vi "Cursor Page.vi"() -> ()   [LabVIEW 2020, in "3D Plot.lvclass"]
uses:
  <vilib>/Math Plots/3D Math Plots/3D Plot/3D Plot/3D Plot.lvclass
  <vilib>/Math Plots/3D Math Plots/3D Plot/3D Plot/Typedef/Cursor Property Array.ctl
  <vilib>/Math Plots/3D Math Plots/3D Plot/3D Plot/Typedef/Cursor Property.ctl
  <vilib>/Math Plots/3D Math Plots/3D Plot/3D Plot/Typedef/Cursor Position.ctl
  <vilib>/Math Plots/3D Math Plots/3D Plot/3D Plot/Typedef/Cursor Point.ctl
  <vilib>/Math Plots/3D Math Plots/3D Plot/3D Plot/Typedef/Sprite Type.ctl
  <vilib>/Math Plots/3D Math Plots/3D Plot/3D Plot/Typedef/Cursor Line.ctl
  <vilib>/Math Plots/3D Math Plots/3D Plot/3D Plot/Typedef/Line Type.ctl
  <vilib>/Math Plots/3D Math Plots/3D Plot/3D Plot/Typedef/Cursor Plane.ctl
  <vilib>/Math Plots/3D Math Plots/3D Plot/3D Plot/Typedef/Cursor Text.ctl
  <vilib>/Math Plots/3D Math Plots/3D Plot/3D Plot/Typedef/Dialog State.ctl
  <vilib>/Math Plots/3D Math Plots/3D Plot/3D Plot/Typedef/Temp Scene State.ctl
  <vilib>/Math Plots/3D Math Plots/3D Plot/3D Plot/Typedef/Temp Scene Property Action.ctl
panel:
  in  "Cursor Name":string="Cursor"
  in  "Plot ID":u16(ring) items=["Plot-1"]
  in  "Name Color":u32(colorbox) caption="Color"
  in  "Background Color":u32(colorbox) caption="Background color"
  in  "Name":u16=1 caption="Size" min=1 step=1
  in  "Show Position":bool caption="Show position"
  in  "Show Name":bool caption="Show name"
  in  "Background Opacity":sgl(slide) caption="Background opacity(%)" min=0 max=100 scale=0.0..100.0
  in  "XY Plane Visible":bool caption="XY plane visible"
  in  "XZ Plane Visible":bool caption="XZ plane visible"
  in  "YZ Plane Visible":bool caption="YZ plane visible"
  in  "Plane Color":u32(colorbox) caption="Plane color"
  in  "Plane Opacity":sgl(slide) caption="Plane opacity(%)" min=0 max=100 scale=0.0..100.0
  in  "X Position":sgl caption="X position"
  in  "Z Position":sgl caption="Z position"
  in  "Y Position":sgl caption="Y position"
  in  "Lock Style":u16(ring) caption="Lock style" items=["Fixed", "Nearest Plot", "Snap to Plot"]
  in  "Cursor Visible":bool caption="Cursor visible"
  in  "Cursor Enable":bool caption="Cursor enable"
  in  "Line Style":u16(ring) caption="Line style"
  in  "Line Color":u32(colorbox) caption="Line color"
  in  "Line Width":sgl=0.001 caption="Line width" min=0.001 step=1
  in  "Point Style":u16(ring) caption="Point style"
  in  "Point Size":sgl=0.001 caption="Point size" min=0.001 step=1
  in  "Point Color":u32(colorbox) caption="Point color"
  in  "Cursor List":i32(listbox) caption="Cursor list"
  in  "New":bool
  in  "Delete":bool
  in  "Move Up":bool caption="Move up"
  in  "Move Down":bool caption="Move down"
  out "Cursor Property Array Out":T1
  in  "Cursor Property Array In":T1
  in  "Event Registration":refnum<event-registration>
  # "Cursor"
  # "Cursor Point"
  # "Cursor Line"
  # "Cursor General"
  # "Cursor Plane"
  # "Cursor Text"
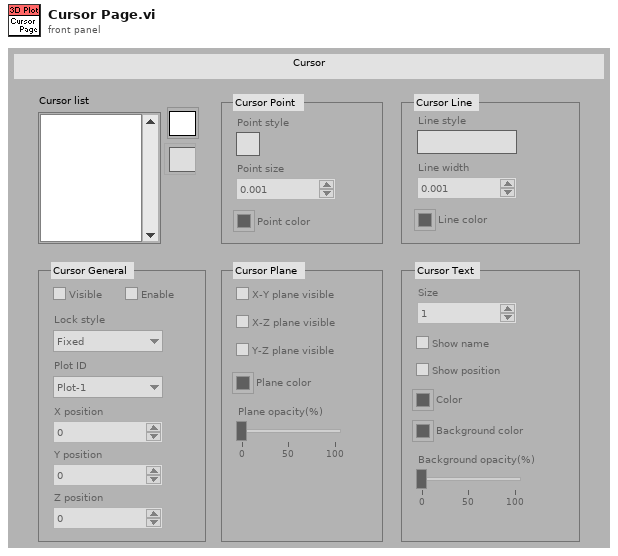
[diagram p1: front panel]
types:
  T1 = typedef "3D Plot.lvclass/Cursor Property Array.ctl" = T2[]
  T2 = typedef "3D Plot.lvclass/Cursor Property.ctl" = cluster{"Cursor Visible":bool, "Cursor Enable":bool, "Cursor Position":T3, "Cursor Point":T4, "Cursor Line":T6, "Cursor Plane":T8, "Cursor Text":T9}
  T3 = typedef "3D Plot.lvclass/Cursor Position.ctl" = cluster{"Cursor Plot ID":i32, "Cursor X":sgl, "Cursor Y":sgl, "Cursor Z":sgl, "Cursor Snap To":enum16{"Fixed", "Nearest Plot", "Snap to Plot"}}
  T4 = typedef "3D Plot.lvclass/Cursor Point.ctl" = cluster{"Cursor Point Color":u32, "Cursor Point Size":sgl, "Cursor Point Style":T5}
  T5 = typedef "3D Plot.lvclass/Sprite Type.ctl" = enum16{"None", "Empty Square", "Solid Square", "Empty Diamond", "Solid Diamond", "Empty Circle", "Solid Circle", "Asterisk", "Bold X", "Wireframe Sphere", "Solid Sphere", "Wireframe Cube", "Solid Cube"}
  T6 = typedef "3D Plot.lvclass/Cursor Line.ctl" = cluster{"Cursor Line Color":u32, "Cursor Line Width":sgl, "Cursor Line Style":T7}
  T7 = typedef "3D Plot.lvclass/Line Type.ctl" = enum16{"None", "Solid", "Dash", "Dot", "Dash Dot"}
  T8 = typedef "3D Plot.lvclass/Cursor Plane.ctl" = cluster{"Cursor Plane Color":u32, "Cursor Plane Opacity":sgl, "Draw Cursor Plane X-Z":bool, "Draw Cursor Plane Y-Z":bool, "Draw Cursor Plane X-Y":bool}
  T9 = typedef "3D Plot.lvclass/Cursor Text.ctl" = cluster{"Cursor Text":string, "Cursor Text Size":u16, "Cursor Show Position":bool, "Cursor Show Name":bool, "Cursor Text Color":u32, "Background Color":u32, "Background Opacity":sgl}
  T10 = typedef "3D Plot.lvclass/Dialog State.ctl" = enum16{"Initialize", "Read Porperty", "Write Property", "Idle", "Exit"}
  T11 = typedef "3D Plot.lvclass/Temp Scene Property Action.ctl" = enum16{"Graph Property", "Light Property", "Axis Property", "Value Pair Property", "Format Property", "Cursor Property", "Plot Specific Property"}
  T12 = typedef "3D Plot.lvclass/Temp Scene State.ctl" = enum16{"Create", "Update Scene", "Get Plot Representation", "Destory"}
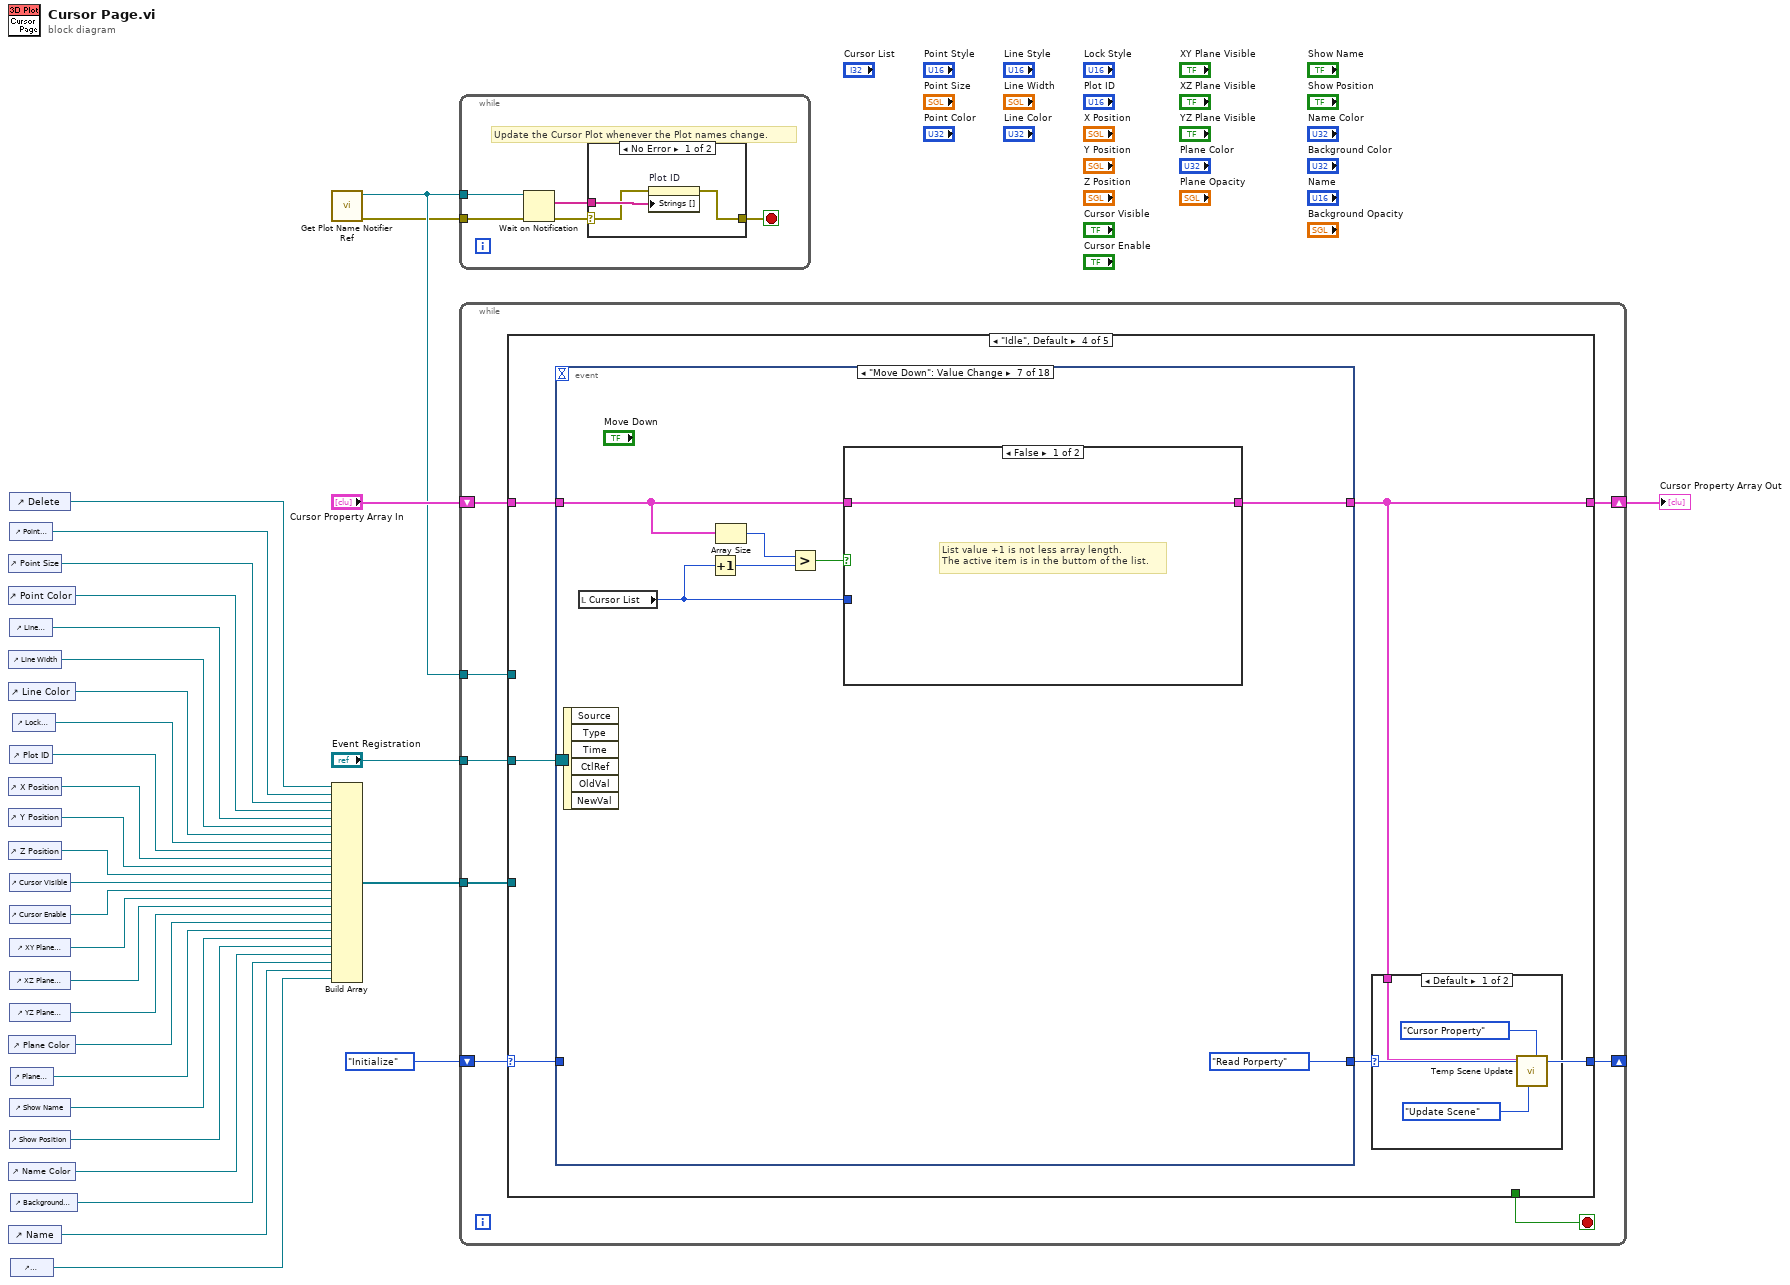
[diagram p0: block diagram]
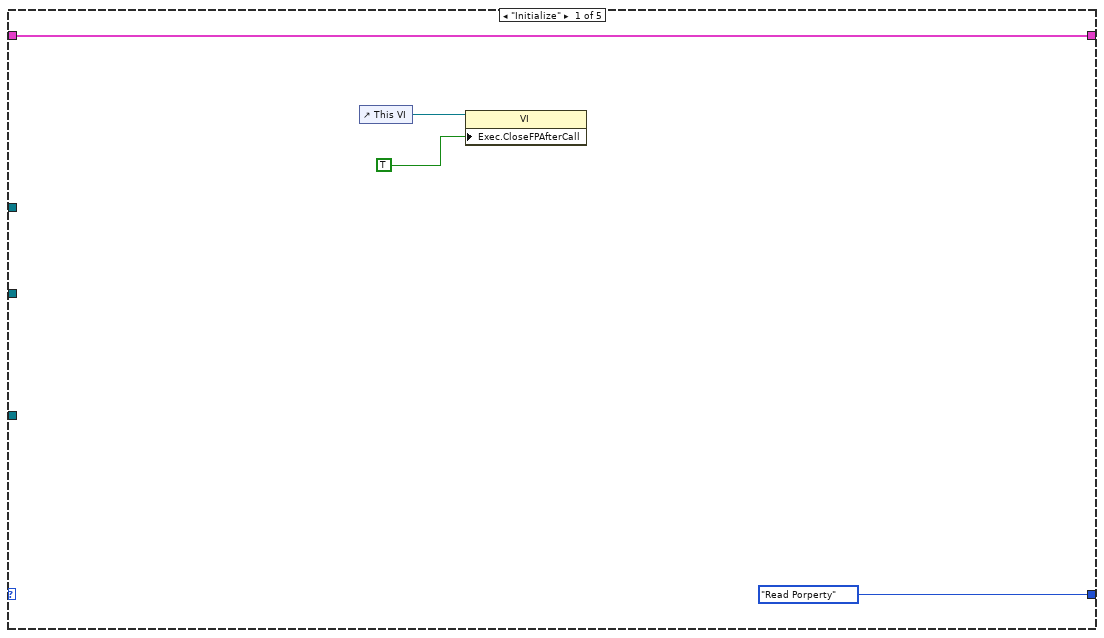
[diagram p3: hidden frame]
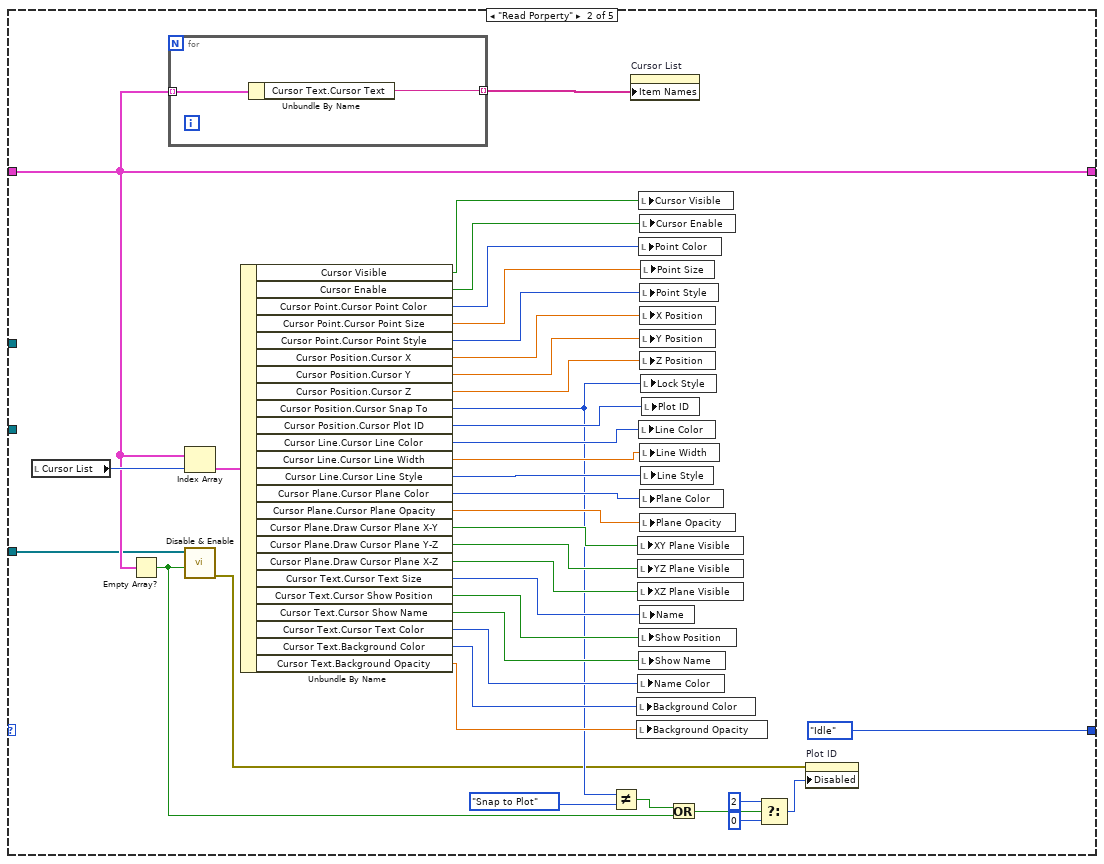
[diagram p4: hidden frame]
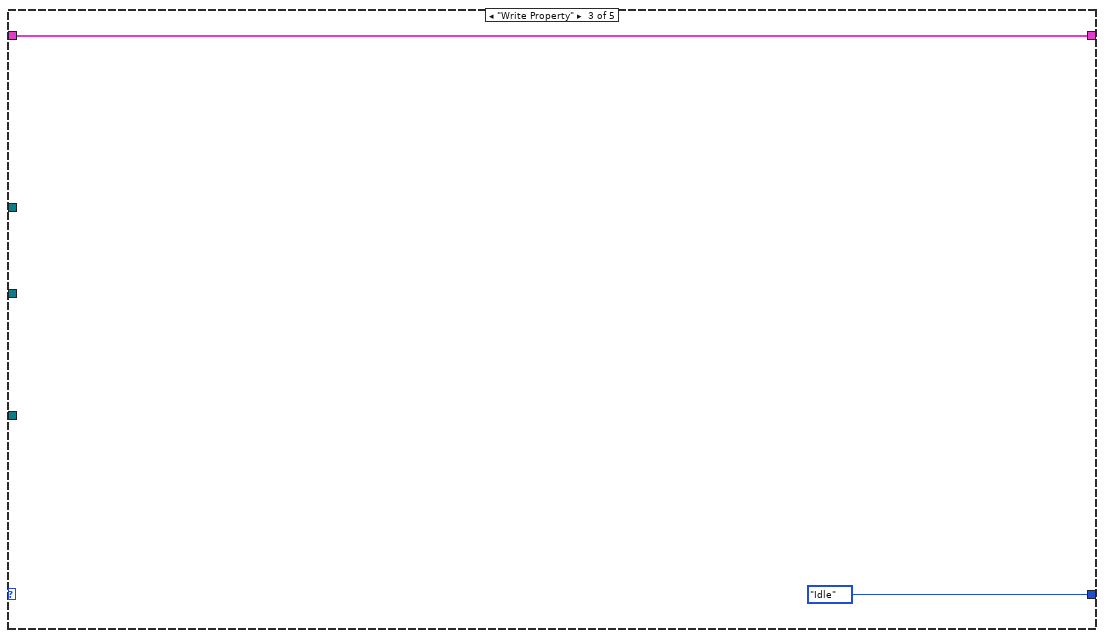
[diagram p5: hidden frame]
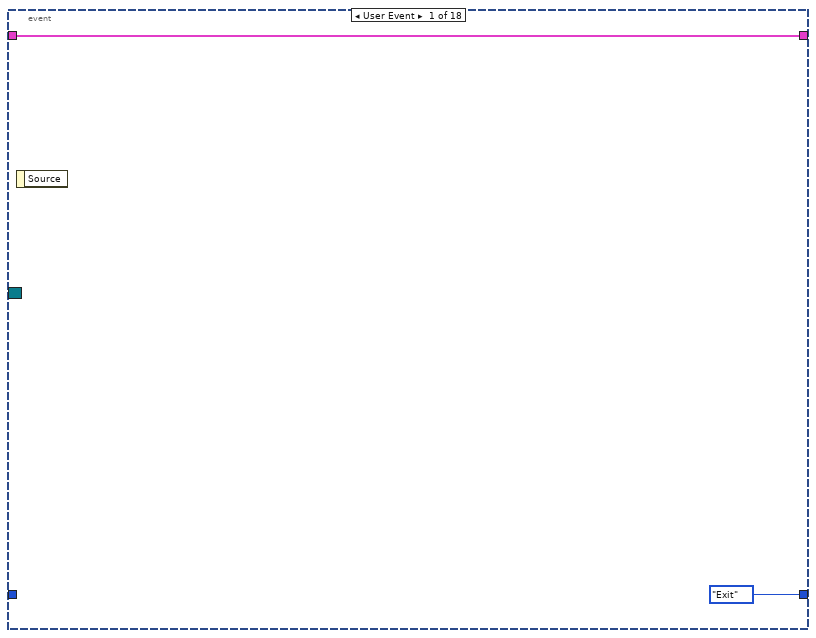
[diagram p7: hidden frame]
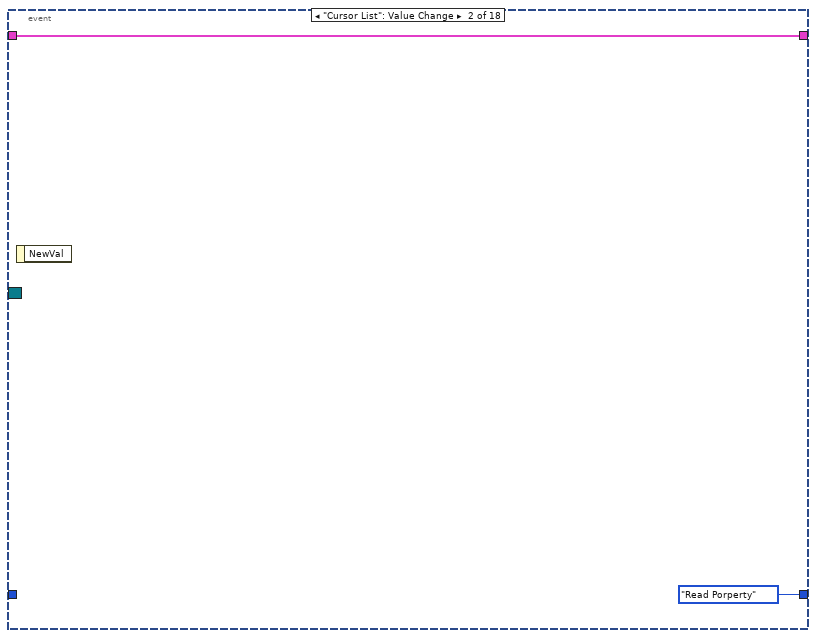
[diagram p8: hidden frame]
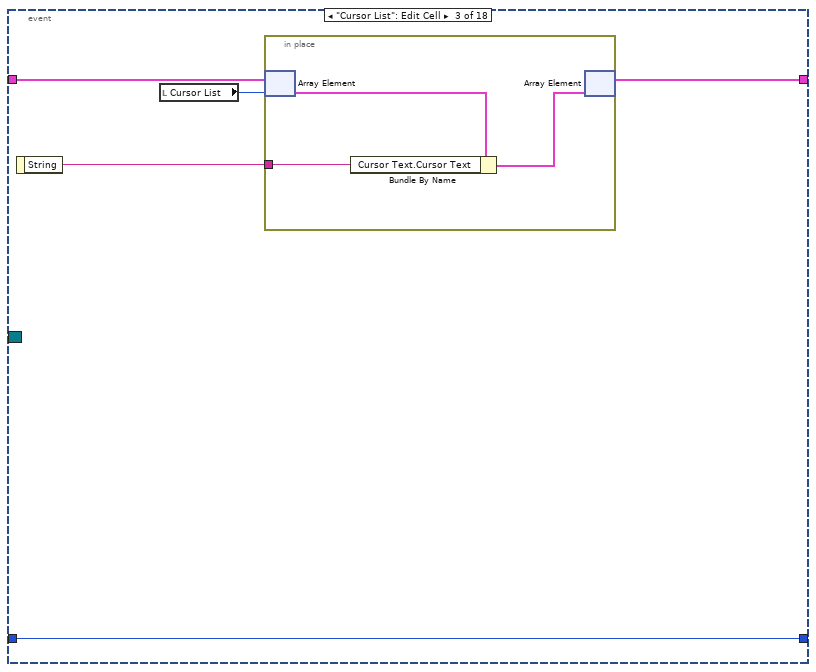
[diagram p9: hidden frame]
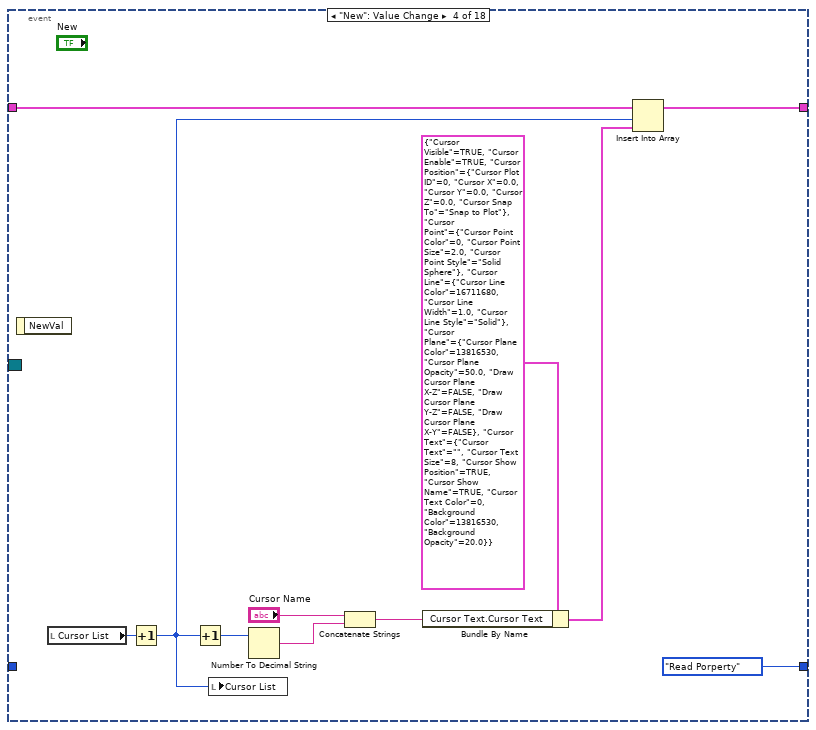
[diagram p10: hidden frame]
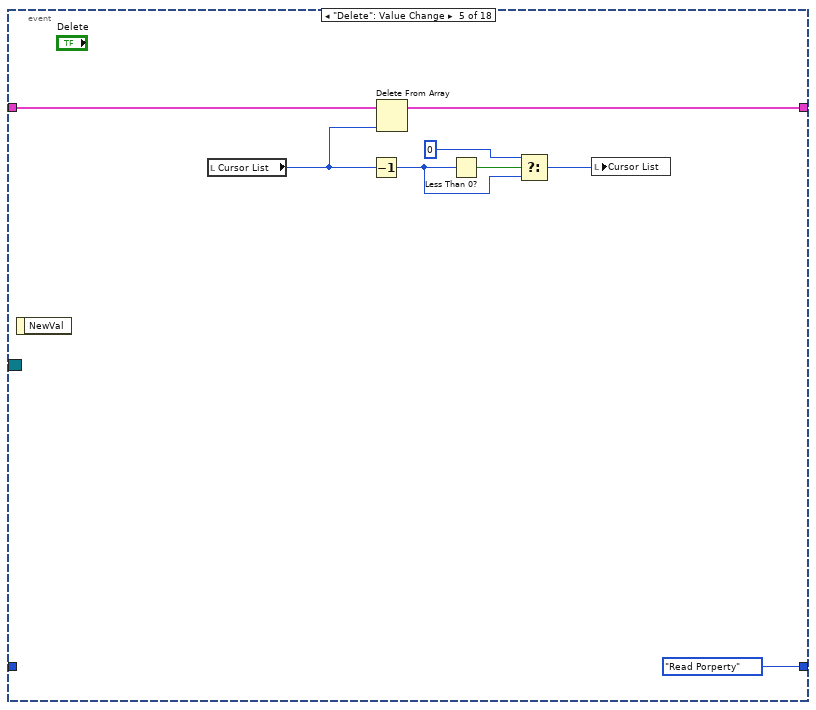
[diagram p11: hidden frame]
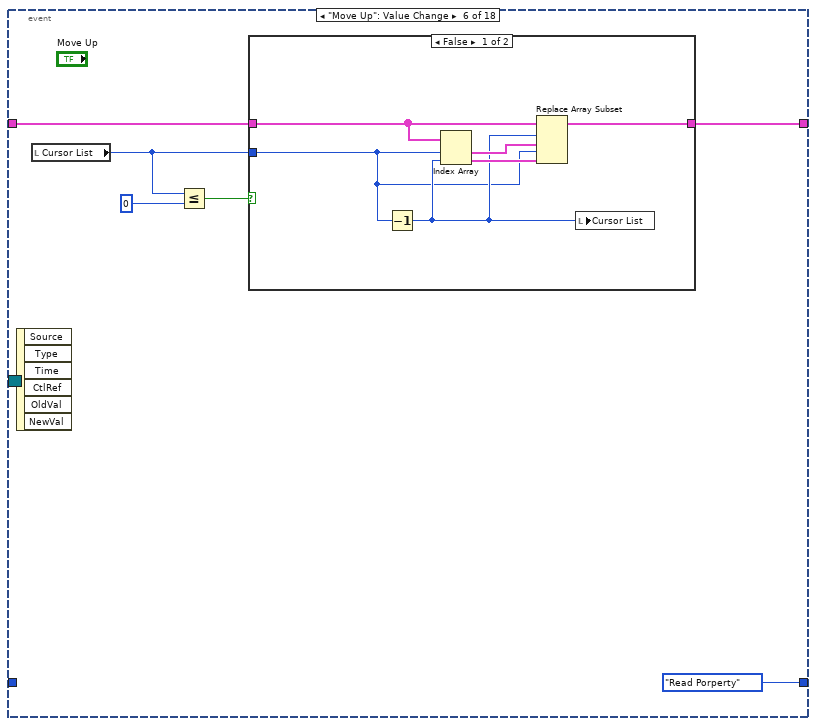
[diagram p12: hidden frame]
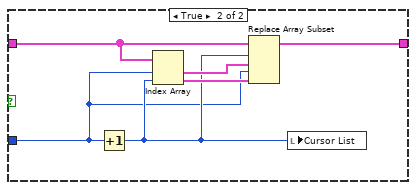
[diagram p14: hidden frame]
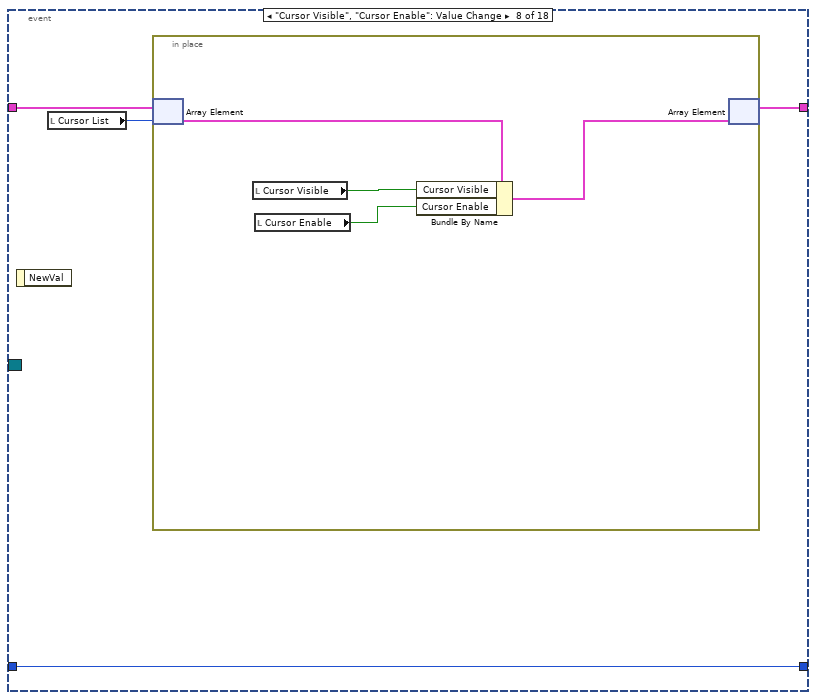
[diagram p15: hidden frame]
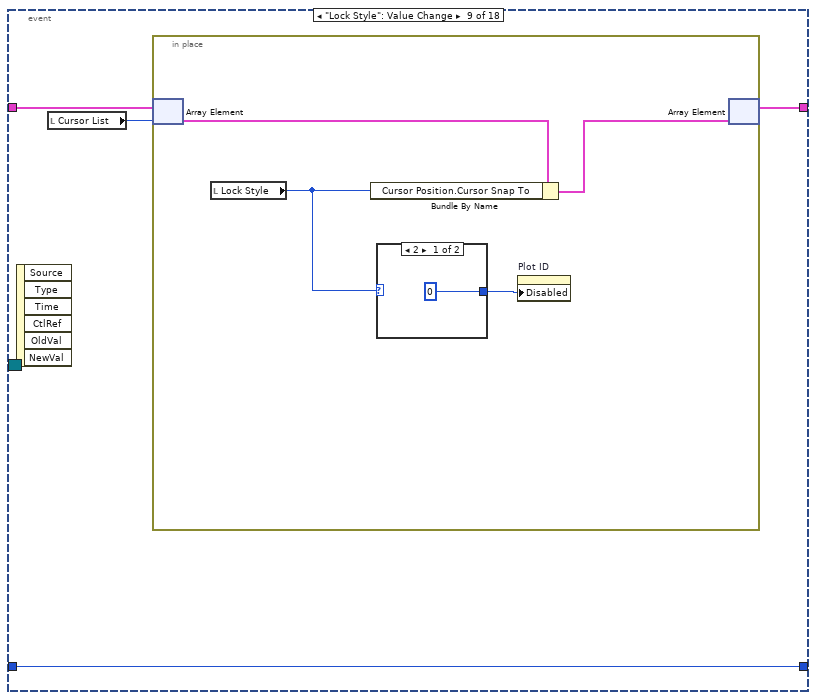
[diagram p16: hidden frame]
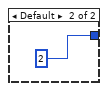
[diagram p17: hidden frame]
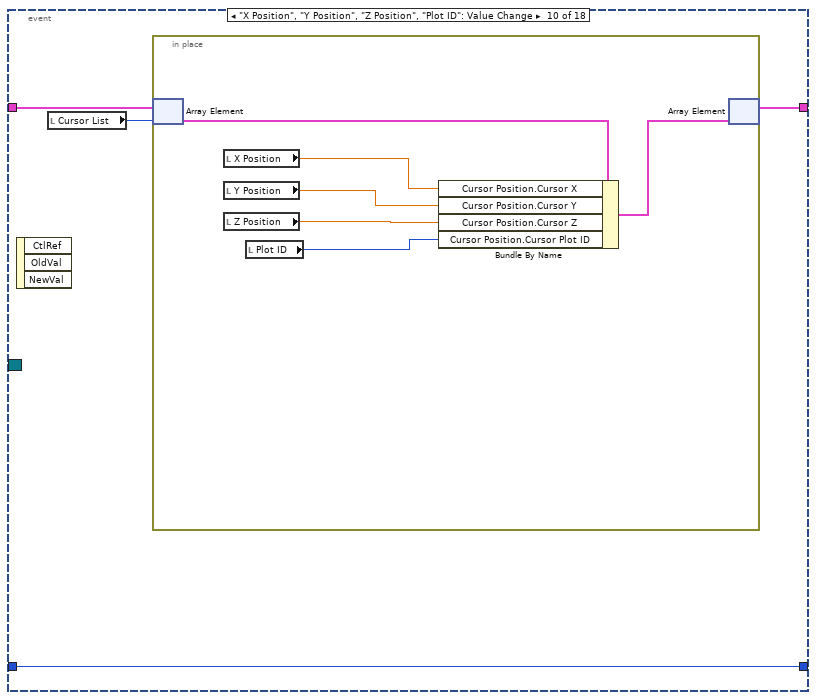
[diagram p18: hidden frame]
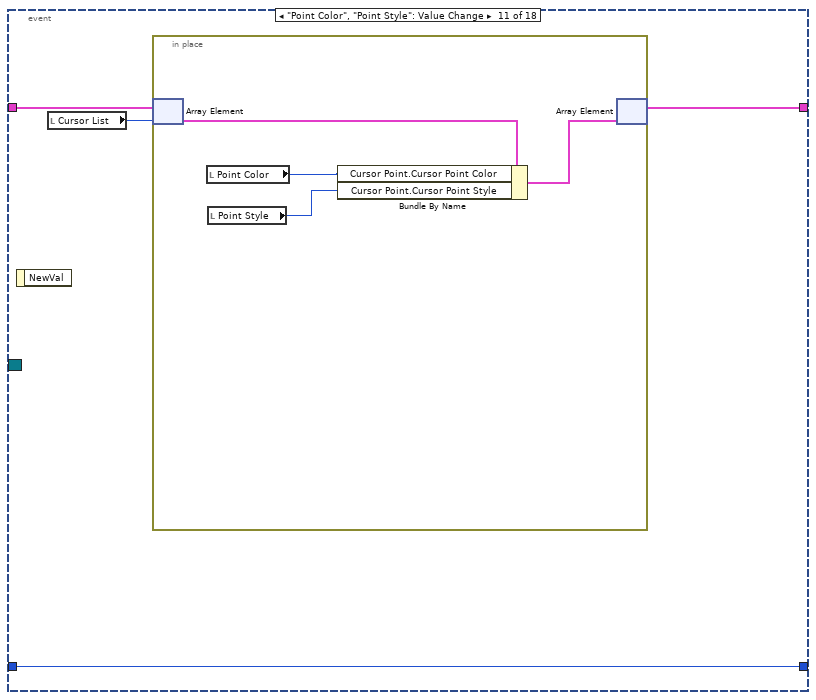
[diagram p19: hidden frame]
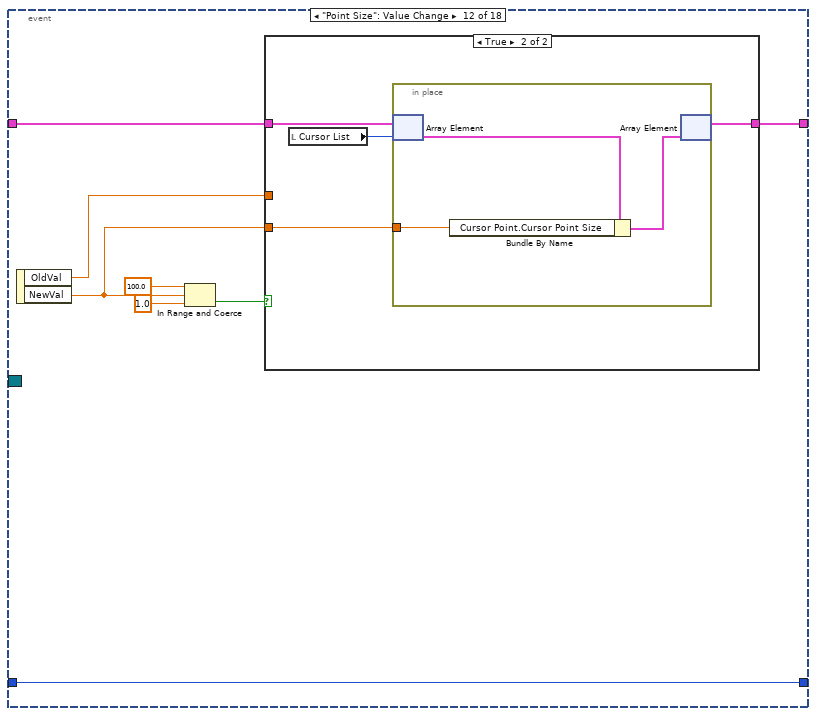
[diagram p20: hidden frame]
diagram:
  n1 = control-ref of="Point Size"() -> (w25:refnum<vi>)
  n2 = control-ref of="Point Color"() -> (w24:refnum<vi>)
  n3 = control-ref of="Line Width"() -> (w22:refnum<vi>)
  n4 = control-ref of="Line Color"() -> (w21:refnum<vi>)
  n5 = control-ref of="X Position"() -> (w18:refnum<vi>)
  n6 = control-ref of="Y Position"() -> (w17:refnum<vi>)
  n7 = control-ref of="Z Position"() -> (w16:refnum<vi>)
  n8 = control-ref of="Plane Color"() -> (w10:refnum<vi>)
  n9 = control-ref of="Name Color"() -> (w7:refnum<vi>)
  n10 = control-ref of="Name"() -> (w5:refnum<vi>)
  n11 = control-ref of="Delete"() -> (w1:refnum<vi>)
  n12 = control-ref of="Point Style"() -> (w26:refnum<vi>)
  n13 = control-ref of="Line Style"() -> (w23:refnum<vi>)
  n14 = control-ref of="Plot ID"() -> (w19:refnum<vi>)
  n15 = control-ref of="Cursor Visible"() -> (w15:refnum<vi>)
  n16 = control-ref of="Cursor Enable"() -> (w14:refnum<vi>)
  n17 = control-ref of="XY Plane Visible"() -> (w13:refnum<vi>)
  n18 = control-ref of="XZ Plane Visible"() -> (w12:refnum<vi>)
  n19 = control-ref of="YZ Plane Visible"() -> (w11:refnum<vi>)
  n20 = control-ref of="Show Name"() -> (w9:refnum<vi>)
  n21 = control-ref of="Show Position"() -> (w8:refnum<vi>)
  n22 = control-ref of="Plane Opacity"() -> (w3:refnum<vi>)
  n23 = control-ref of="Background Color"() -> (w6:refnum<vi>)
  n24 = control-ref of="Background Opacity"() -> (w4:refnum<vi>)
  n25 = control-ref of="Lock Style"() -> (w20:refnum<vi>)
  n26 = call <vilib>:"Get Plot Name Notifier Ref.vi"() -> ("error out"=w27:errorcluster, "Plot Names Notifier Ref"=w28:refnum<notifier>)  [unwired: 1 in, 9 out]
  n27 = Build Array(w1, w26, w25, w24, w23, w22, w21, w20, w19, w18, w17, w16, w15, w14, w13, w12, w11, w10, w3, w9, w8, w7, w6, w5, w4) -> (w2:refnum<vi>[])
  n28 = while {
    tunnel: w28 -> [w37]
    tunnel: w27 -> [w33]
    stop <- w34 stop-if-true
    # "Update the Cursor Plot whenever the Plot names change."
    n29 = Wait on Notification(notifier=w37, error in (no error)=w33) -> (notification=w36:string[], error out=w35:errorcluster)  [unwired: 4 out]
    n30 = case shown="No Error" w35 {
      selector: w35 -> [w39 w41]
      tunnel: w36 -> [w40 _]
      tunnel: [w38 w41] -> w34
      frame No Error {
        n31 = property on="Plot ID" class="Ring (strict)"(error in=w39, "Strings []"=w40) -> (error out=w38:errorcluster)  [unwired: 1 in, 1 out]
      }
      frame Error {
      }
    }
  }
  n32 = while {
    shift-right: [w48] -> w32
    shift-left: "Cursor Property Array In" -> [w49]
    shift-right: [w44] -> _
    shift-left: Dialog_State."Initialize" -> [w47]
    tunnel: "Event Registration" -> [w45]
    tunnel: w28 -> [w43]
    tunnel: w2 -> [w42]
    stop <- w46 stop-if-true
    n33 = case shown="\"Idle\", Default" w47 {
      selector: w47 -> [_ _ _ w98 _]
      tunnel: w49 -> [w52 w64 w94 w100 w279]
      tunnel: [w52 w64 w94 w97 w279] -> w48
      tunnel: [Dialog_State."Read Porperty" Dialog_State."Idle" Dialog_State."Idle" w96 Dialog_State."Exit"] -> w44
      tunnel: [_ _ _ _ TRUE] -> w46
      tunnel: w45 -> [_ _ _ w99 _]
      tunnel: w43 -> [_ _ _ _ w278]
      tunnel: w42 -> [_ w63 _ _ _]
      frame "Initialize" {
        n34 = control-ref of="This VI"() -> (w51:refnum<vi>)
        n35 = property class="VI"(reference=w51, "Exec.CloseFPAfterCall"=TRUE ("Execution:Close After Call")) -> ()  [unwired: 1 in, 2 out]
      }
      frame "Read Porperty" {
        n36 = local read "Cursor List"() -> (w66:i32)
        n37 = Empty Array?(array=w64) -> (empty?=w59:bool)
        n38 = for {
          tunnel: w64 -> [w93] mode=indexing
          tunnel: [w92] -> w67 mode=indexing
          n39 = Unbundle By Name(w93) -> ("Cursor Text.Cursor Text"=w92:string)
        }
        n40 = Index Array(array=w64, index=w66) -> (element=w90:T2)
        n41 = call <vilib>:"Disable & Enable.vi"("Disabled?"=w59, "Control Ref Array"=w63) -> ("error out"=w54:errorcluster)  [unwired: 1 in, 8 out]
        n42 = Unbundle By Name(w90) -> ("Cursor Visible"=w89:bool, "Cursor Enable"=w88:bool, "Cursor Point.Cursor Point Color"=w87:u32, "Cursor Point.Cursor Point Size"=w86:sgl, "Cursor Point.Cursor Point Style"=w85:T5, "Cursor Position.Cursor X"=w84:sgl, "Cursor Position.Cursor Y"=w83:sgl, "Cursor Position.Cursor Z"=w82:sgl, "Cursor Position.Cursor Snap To"=w61:enum16{"Fixed", "Nearest Plot", "Snap to Plot"}, "Cursor Position.Cursor Plot ID"=w65:i32, "Cursor Line.Cursor Line Color"=w81:u32, "Cursor Line.Cursor Line Width"=w80:sgl, "Cursor Line.Cursor Line Style"=w79:T7, "Cursor Plane.Cursor Plane Color"=w78:u32, "Cursor Plane.Cursor Plane Opacity"=w77:sgl, "Cursor Plane.Draw Cursor Plane X-Y"=w76:bool, "Cursor Plane.Draw Cursor Plane Y-Z"=w75:bool, "Cursor Plane.Draw Cursor Plane X-Z"=w74:bool, "Cursor Text.Cursor Text Size"=w70:u16, "Cursor Text.Cursor Show Position"=w72:bool, "Cursor Text.Cursor Show Name"=w73:bool, "Cursor Text.Cursor Text Color"=w69:u32, "Cursor Text.Background Color"=w71:u32, "Cursor Text.Background Opacity"=w68:sgl)
        n43 = Not Equal?(x=w61, y=enum16{"Fixed", "Nearest Plot", "Snap to Plot"}."Snap to Plot" ("Cursor Position.Cursor Snap To")) -> (x != y?=w60:bool)
        n44 = property on="Cursor List" class="LstBox (strict)"("Item Names"=w67) -> ()  [unwired: 2 in, 2 out]
        n45 = local write "Background Color"(w71) -> ()
        n46 = local write "Background Opacity"(w68) -> ()
        n47 = local write "XY Plane Visible"(w76) -> ()
        n48 = local write "YZ Plane Visible"(w75) -> ()
        n49 = local write "XZ Plane Visible"(w74) -> ()
        n50 = local write "Name Color"(w69) -> ()
        n51 = local write "Cursor Visible"(w89) -> ()
        n52 = local write "Point Color"(w87) -> ()
        n53 = local write "Line Color"(w81) -> ()
        n54 = local write "Show Position"(w72) -> ()
        n55 = local write "Show Name"(w73) -> ()
        n56 = local write "Cursor Enable"(w88) -> ()
        n57 = local write "Point Style"(w85) -> ()
        n58 = local write "X Position"(w84) -> ()
        n59 = local write "Y Position"(w83) -> ()
        n60 = local write "Z Position"(w82) -> ()
        n61 = local write "Line Width"(w80) -> ()
        n62 = local write "Plane Color"(w78) -> ()
        n63 = local write "Plane Opacity"(w77) -> ()
        n64 = local write "Name"(w70) -> ()
        n65 = local write "Point Size"(w86) -> ()
        n66 = local write "Lock Style"(w61) -> ()
        n67 = local write "Line Style"(w79) -> ()
        n68 = local write "Plot ID"(w65) -> ()
        n69 = Or(x=w60, y=w59) -> (x .or. y?=w56:bool)
        n70 = Select(t=u8 2 ("Disabled"), s=w56, f=u8 0 ("Disabled")) -> (s? t:f=w55:u8)
        n71 = property on="Plot ID" class="Ring (strict)"(error in=w54, "Disabled"=w55) -> ()  [unwired: 1 in, 2 out]
      }
      frame "Write Property" {
      }
      frame "Idle", Default {
        n72 = event shown="[6] \"Move Down\": Value Change" {
          selector: w99 -> [_ _ _ _ _ _ _ _ _ _ _ _ _ _ _ _ _ _]
          dyn-events: _ -> [_ _ _ _ _ _ _ _ _ _ _ _ _ _ _ _ _ _]
          timeout: _ -> [_ _ _ _ _ _ _ _ _ _ _ _ _ _ _ _ _ _]
          tunnel: w100 -> [w105 w107 w112 w126 w134 w140 w150 w165 w173 w182 w193 w205 w218 w227 w243 w254 w261 w273]
          tunnel: [w105 w107 w109 w125 w133 w139 w154 w164 w172 w181 w192 w204 w216 w226 w242 w253 w260 w272] -> w97
          tunnel: [Dialog_State."Exit" Dialog_State."Read Porperty" w108 Dialog_State."Read Porperty" Dialog_State."Read Porperty" Dialog_State."Read Porperty" Dialog_State."Read Porperty" w162 w170 w180 w190 w203 w215 w223 w240 w251 w258 w270] -> w96
          tunnel: w98 -> [_ _ w108 _ _ _ _ w162 w170 w180 w190 w203 w215 w223 w240 w251 w258 w270]
          event User Event {
            n73 = event-data() -> ()  [unwired: 2 out]
          }
          event "Cursor List": Value Change {
            n74 = event-data() -> ()  [unwired: 2 out]
          }
          event "Cursor List": Edit Cell {
            n75 = event-data() -> ("String"=w110:string)  [unwired: 1 out]
            n76 = local read "Cursor List"() -> (w111:i32)
            n77 = in-place {
              in-place-border: w110 -> [w113]
              n78 = in-place-array #1(w112, w111) -> (w115:T2)
              n79 = Bundle By Name(cluster=w115, "Cursor Text.Cursor Text"=w113) -> (w114:T2)
              n80 = in-place-array #1(w114) -> (w109:T1)  [unwired: 1 out]
            }
          }
          event "New": Value Change {
            n81 = event-data() -> ()  [unwired: 2 out]
            n82 = local read "Cursor List"() -> (w117:i32)
            n83 = Increment(x=w117) -> (x+1=w116:i32)
            n84 = Increment(x=w116) -> (x+1=w118:i32)
            n85 = local write "Cursor List"(w116) -> ()
            n86 = Number To Decimal String(number=w118) -> (decimal integer string=w120:string)  [unwired: 1 out]
            n87 = Concatenate Strings("Cursor Name", w120) -> (w122:string)
            n88 = Bundle By Name(cluster=T2 {"Cursor Visible"=TRUE, "Cursor Enable"=TRUE, "Cursor Position"={"Cursor Plot ID"=0, "Cursor X"=0.0, "Cursor Y"=0.0, "Cursor Z"=0.0, "Cursor Snap To"=enum."Snap to Plot"}, "Cursor Point"={"Cursor Point Color"=0, "Cursor Point Size"=2.0, "Cursor Point Style"=enum."Solid Sphere"}, "Cursor Line"={"Cursor Line Color"=16711680, "Cursor Line Width"=1.0, "Cursor Line Style"=enum."Solid"}, "Cursor Plane"={"Cursor Plane Color"=13816530, "Cursor Plane Opacity"=50.0, "Draw Cursor Plane X-Z"=FALSE, "Draw Cursor Plane Y-Z"=FALSE, "Draw Cursor Plane X-Y"=FALSE}, "Cursor Text"={"Cursor Text"="", "Cursor Text Size"=8, "Cursor Show Position"=TRUE, "Cursor Show Name"=TRUE, "Cursor Text Color"=0, "Background Color"=13816530, "Background Opacity"=20.0}} ("new element/subarray"), "Cursor Text.Cursor Text"=w122) -> (w123:T2)
            n89 = Insert Into Array(array=w126, index=w116, new element=w123) -> (w125:T1)
          }
          event "Delete": Value Change {
            n90 = event-data() -> ()  [unwired: 2 out]
            n91 = local read "Cursor List"() -> (w128:i32)
            n92 = Decrement(x=w128) -> (x-1=w129:i32)
            n93 = Delete From Array(array=w134, index=w128) -> (array with subset deleted=w133:T1)  [unwired: 1 in, 1 out]
            n94 = Less Than 0?(x=w129) -> (x < 0?=w131:bool)
            n95 = Select(t=0, s=w131, f=w129) -> (s? t:f=w127:i32)
            n96 = local write "Cursor List"(w127) -> ()
          }
          event "Move Up": Value Change {
            n97 = event-data() -> ()  [unwired: 7 out]
            n98 = local read "Cursor List"() -> (w135:i32)
            n99 = Less Or Equal?(x=w135, y=0) -> (x <= y?=w136:bool)
            n100 = case shown="False" w136 {
              tunnel: w140 -> [w144 w147]
              tunnel: [w143 w147] -> w139
              tunnel: w135 -> [w141 _]
              frame False {
                n101 = Decrement(x=w141) -> (x-1=w142:i32)
                n102 = Index Array(array=w144, index #1=w141, index #2=w142) -> (element #1=w145:T2, element #2=w146:T2)
                n103 = Replace Array Subset(array=w144, new element #1=w145, index #1=w142, new element #2=w146, index #2=w141) -> (w143:T1)
                n104 = local write "Cursor List"(w142) -> ()
              }
              frame True {
                # "List value is less or equal to 0.\nThe active item is in the top of the list."
              }
            }
          }
          event "Move Down": Value Change {
            n105 = event-data() -> ()  [unwired: 7 out]
            n106 = local read "Cursor List"() -> (w149:i32)
            n107 = Increment(x=w149) -> (x+1=w152:i32)
            n108 = Array Size(array=w150) -> (size(s)=w151:i32)
            n109 = Greater?(x=w151, y=w152) -> (0:w148:bool)
            n110 = case shown="False" w148 {
              tunnel: [w155 w159] -> w154
              tunnel: w150 -> [w155 w157]
              tunnel: w149 -> [_ w156]
              frame False {
                # "List value +1 is not less array length.\nThe active item is in the buttom of the list."
              }
              frame True {
                n111 = Increment(x=w156) -> (x+1=w158:i32)
                n112 = Index Array(array=w157, index #1=w156, index #2=w158) -> (element #1=w160:T2, element #2=w161:T2)
                n113 = Replace Array Subset(array=w157, new element #1=w160, index #1=w158, new element #2=w161, index #2=w156) -> (w159:T1)
                n114 = local write "Cursor List"(w158) -> ()
              }
            }
          }
          event "Cursor Visible", "Cursor Enable": Value Change {
            n115 = event-data() -> ()  [unwired: 2 out]
            n116 = local read "Cursor List"() -> (w163:i32)
            n117 = in-place {
              n118 = in-place-array #2(w165, w163) -> (w167:T2)
              n119 = local read "Cursor Visible"() -> (w169:bool)
              n120 = local read "Cursor Enable"() -> (w168:bool)
              n121 = Bundle By Name(cluster=w167, "Cursor Visible"=w169, "Cursor Enable"=w168) -> (w166:T2)
              n122 = in-place-array #2(w166) -> (w164:T1)  [unwired: 1 out]
            }
          }
          event "Lock Style": Value Change {
            n123 = event-data() -> ()  [unwired: 7 out]
            n124 = local read "Cursor List"() -> (w171:i32)
            n125 = in-place {
              n126 = in-place-array #3(w173, w171) -> (w177:T2)
              n127 = local read "Lock Style"() -> (w175:u16)
              n128 = Bundle By Name(cluster=w177, "Cursor Position.Cursor Snap To"=w175) -> (w176:T2)
              n129 = case shown="2" w175 {
                tunnel: [u8 0 ("Disabled") u8 2 ("Disabled")] -> w174
                frame 2 {
                }
                frame Default {
                }
              }
              n130 = property on="Plot ID" class="Ring (strict)"("Disabled"=w174) -> ()  [unwired: 2 in, 2 out]
              n131 = in-place-array #3(w176) -> (w172:T1)  [unwired: 1 out]
            }
          }
          event "X Position", "Y Position", "Z Position", "Plot ID": Value Change {
            n132 = event-data() -> ()  [unwired: 4 out]
            n133 = local read "Cursor List"() -> (w183:i32)
            n134 = in-place {
              n135 = in-place-array #4(w182, w183) -> (w189:T2)
              n136 = local read "X Position"() -> (w187:sgl)
              n137 = local read "Y Position"() -> (w186:sgl)
              n138 = local read "Z Position"() -> (w185:sgl)
              n139 = local read "Plot ID"() -> (w184:u16)
              n140 = Bundle By Name(cluster=w189, "Cursor Position.Cursor X"=w187, "Cursor Position.Cursor Y"=w186, "Cursor Position.Cursor Z"=w185, "Cursor Position.Cursor Plot ID"=w184) -> (w188:T2)
              n141 = in-place-array #4(w188) -> (w181:T1)  [unwired: 1 out]
            }
          }
          event "Point Color", "Point Style": Value Change {
            n142 = event-data() -> ()  [unwired: 2 out]
            n143 = local read "Cursor List"() -> (w191:i32)
            n144 = in-place {
              n145 = in-place-array #5(w193, w191) -> (w196:T2)
              n146 = local read "Point Color"() -> (w197:u32)
              n147 = local read "Point Style"() -> (w194:u16)
              n148 = Bundle By Name(cluster=w196, "Cursor Point.Cursor Point Color"=w197, "Cursor Point.Cursor Point Style"=w194) -> (w195:T2)
              n149 = in-place-array #5(w195) -> (w192:T1)  [unwired: 1 out]
            }
          }
          event "Point Size": Value Change {
            n150 = event-data() -> ("OldVal"=w198:sgl, "NewVal"=w199:sgl)  [unwired: 1 out]
            n151 = In Range and Coerce(upper limit=sgl 100.0, x=w199, lower limit=sgl 1.0) -> (In Range?=w200:bool)  [unwired: 1 out]
            n152 = case shown="True" w200 {
              tunnel: w205 -> [w206 w211]
              tunnel: [w206 w210] -> w204
              tunnel: w199 -> [_ w208]
              tunnel: w198 -> [w207 _]
              frame False {
                n153 = local write "Point Size"(w207) -> ()
              }
              frame True {
                n154 = local read "Cursor List"() -> (w209:i32)
                n155 = in-place {
                  in-place-border: w208 -> [w212]
                  n156 = in-place-array #6(w211, w209) -> (w214:T2)
                  n157 = Bundle By Name(cluster=w214, "Cursor Point.Cursor Point Size"=w212) -> (w213:T2)
                  n158 = in-place-array #6(w213) -> (w210:T1)  [unwired: 1 out]
                }
              }
            }
          }
          event "Line Color", "Line Style": Value Change {
            n159 = event-data() -> ()  [unwired: 2 out]
            n160 = local read "Cursor List"() -> (w217:i32)
            n161 = in-place {
              n162 = in-place-array #7(w218, w217) -> (w222:T2)
              n163 = local read "Line Color"() -> (w220:u32)
              n164 = local read "Line Style"() -> (w219:u16)
              n165 = Bundle By Name(cluster=w222, "Cursor Line.Cursor Line Color"=w220, "Cursor Line.Cursor Line Style"=w219) -> (w221:T2)
              n166 = in-place-array #7(w221) -> (w216:T1)  [unwired: 1 out]
            }
          }
          event "Line Width": Value Change {
            n167 = event-data() -> ("OldVal"=w224:sgl, "NewVal"=w225:sgl)  [unwired: 1 out]
            n168 = In Range and Coerce(upper limit=sgl 100.0, x=w225, lower limit=sgl 1.0) -> (In Range?=w228:bool)  [unwired: 1 out]
            n169 = case shown="True" w228 {
              tunnel: w227 -> [w231 w236]
              tunnel: [w231 w235] -> w226
              tunnel: w225 -> [_ w233]
              tunnel: w224 -> [w232 _]
              frame False {
                n170 = local write "Line Width"(w232) -> ()
              }
              frame True {
                n171 = local read "Cursor List"() -> (w234:i32)
                n172 = in-place {
                  in-place-border: w233 -> [w237]
                  n173 = in-place-array #8(w236, w234) -> (w239:T2)
                  n174 = Bundle By Name(cluster=w239, "Cursor Line.Cursor Line Width"=w237) -> (w238:T2)
                  n175 = in-place-array #8(w238) -> (w235:T1)  [unwired: 1 out]
                }
              }
            }
          }
          event "Plane Color", "XY Plane Visible", "YZ Plane Visible", "XZ Plane Visible": Value Change {
            n176 = event-data() -> ()  [unwired: 2 out]
            n177 = local read "Cursor List"() -> (w241:i32)
            n178 = in-place {
              n179 = in-place-array #9(w243, w241) -> (w249:T2)
              n180 = local read "XY Plane Visible"() -> (w246:bool)
              n181 = local read "XZ Plane Visible"() -> (w244:bool)
              n182 = local read "YZ Plane Visible"() -> (w245:bool)
              n183 = local read "Plane Color"() -> (w247:u32)
              n184 = Bundle By Name(cluster=w249, "Cursor Plane.Cursor Plane Color"=w247, "Cursor Plane.Draw Cursor Plane X-Y"=w246, "Cursor Plane.Draw Cursor Plane X-Z"=w244, "Cursor Plane.Draw Cursor Plane Y-Z"=w245) -> (w248:T2)
              n185 = in-place-array #9(w248) -> (w242:T1)  [unwired: 1 out]
            }
          }
          event "Plane Opacity": Value Change {
            n186 = event-data() -> ("NewVal"=w252:sgl)  [unwired: 1 out]
            n187 = local read "Cursor List"() -> (w250:i32)
            n188 = in-place {
              in-place-border: w252 -> [w255]
              n189 = in-place-array #10(w254, w250) -> (w257:T2)
              n190 = Bundle By Name(cluster=w257, "Cursor Plane.Cursor Plane Opacity"=w255) -> (w256:T2)
              n191 = in-place-array #10(w256) -> (w253:T1)  [unwired: 1 out]
            }
          }
          event "Name Color", "Name", "Show Position", "Show Name", "Background Color": Value Change {
            n192 = event-data() -> ()  [unwired: 2 out]
            n193 = local read "Cursor List"() -> (w259:i32)
            n194 = in-place {
              n195 = in-place-array #11(w261, w259) -> (w268:T2)
              n196 = local read "Name Color"() -> (w266:u32)
              n197 = local read "Background Color"() -> (w263:u32)
              n198 = local read "Show Position"() -> (w264:bool)
              n199 = local read "Show Name"() -> (w262:bool)
              n200 = local read "Name"() -> (w265:u16)
              n201 = Bundle By Name(cluster=w268, "Cursor Text.Cursor Text Color"=w266, "Cursor Text.Cursor Text Size"=w265, "Cursor Text.Cursor Show Position"=w264, "Cursor Text.Cursor Show Name"=w262, "Cursor Text.Background Color"=w263) -> (w267:T2)
              n202 = in-place-array #11(w267) -> (w260:T1)  [unwired: 1 out]
            }
          }
          event "Background Opacity": Value Change {
            n203 = event-data() -> ("NewVal"=w271:sgl)  [unwired: 1 out]
            n204 = local read "Cursor List"() -> (w269:i32)
            n205 = in-place {
              in-place-border: w271 -> [w274]
              n206 = in-place-array #12(w273, w269) -> (w276:T2)
              n207 = Bundle By Name(cluster=w276, "Cursor Text.Background Opacity"=w274) -> (w275:T2)
              n208 = in-place-array #12(w275) -> (w272:T1)  [unwired: 1 out]
            }
          }
        }
        n209 = case shown="Default" w96 {
          tunnel: w97 -> [w101 _]
          frame Default {
            n210 = call <vilib>:"Temp Scene Update.vi"("Property Name"=Temp_Scene_Property_Action."Cursor Property", "State"=Temp_Scene_State."Update Scene", "Property In"=w101) -> ()  [unwired: 3 in, 6 out]
          }
          frame "Exit" {
          }
        }
      }
      frame "Exit" {
        n211 = Release Notifier(notifier=w278, force destroy? (F)=TRUE) -> ()  [unwired: 1 in, 3 out]
      }
    }
  }
  "Cursor Property Array Out" <- w32
